vi "EstimateAbsoluteOrientation2D.vi"(5 "Point Set Weights (Default: Empty - Equal Weights)":dbl[](array[numeric]), 7 "Termination Criterion in":refnum<class "Termination Criteria.lvclass">, 8 "error in":errorcluster, 10 "Reference Point Set (Default - Use First  Set of Corresponding Points Array)":map{i32, T1}(c390), 11 "Image Point Sets":map{i32, T1}[](array[numeric])) -> (0 "error out":errorcluster, 1 "T Vectors":T1[](array[typedef]), 2 "R Matricies":dbl[][][](array[numeric]), 3 "Optimized Points":map{i32, T1}(c390), 4 "Scale Values":dbl[](array[numeric]))   [LabVIEW 2020, in "ar.lvlib"]
doc: "Estimate the Absolute Orientation of multiple views of the same 2D Point Set. \n\nThis can be used to combine multiple samples of the same object point sets to reduce mean square errors in an absolute set of positions."
uses:
  ar.lvlib
  common/Termination Criteria/Termination Criteria.lvclass
  common/Image Point (Float).ctl
  common/Termination Criteria/Termination Criteria.lvclass/Termination Criteria.ctl
  808428ba-76ae-4f0f-a703-b2147cff2032.vi
  EstimateTransformParametersBetweenPointSets.vi
  OptimizePointSetFromPointSetCorrespondenceTransforms.vi
  Dimensions.vi
  common/Termination Criteria/Get Values.vi
  808428ba-76ae-4f0f-a703-b2147cff2032.vi/b761b6b4-53cc-4592-85b1-23315e9e6a73.vi
  SubtractMeanFromPoints.vi
  CovarianceofPointSetsA&B.vi
  DecomposeCovarianceOfPointSetsA&B.vi
  <vilib>/Analysis/baseanly.llb/A x Vector.vi
  <vilib>/Analysis/baseanly.llb/A x B.vi
  <vilib>/Analysis/baseanly.llb/Mean.vi
  <vilib>/Analysis/baseanly.llb/Mean (DBL).vi
  <vilib>/Analysis/baseanly.llb/Real A x B.vi
  <vilib>/Analysis/baseanly.llb/Determinant.vi
  <vilib>/Analysis/baseanly.llb/Real Determinant.vi
  SVDForPointSetCovarainces.vi
  <vilib>/Analysis/_algsub.llb/Matrix Rank.vi
  <vilib>/Analysis/_algsub.llb/Real Matrix Rank.vi
  <vilib>/Analysis/_algsub.llb/Trace.vi
  <vilib>/Analysis/_algsub.llb/Real Matrix Trace.vi
  <vilib>/Utility/error.llb/Error Cluster From Error Code.vi
  <vilib>/Analysis/7linalg.llb/Create Special Real Matrix.vi
  <vilib>/Analysis/Matrix/Numeric/Conversions/Array To Matrix - RA2.vi
  <vilib>/Analysis/7linalg.llb/SVD Decomposition.vi
  <vilib>/Analysis/7linalg.llb/Real SVD Decomposition.vi
  <vilib>/Analysis/7linalg.llb/Create Special Matrix.vi
  <vilib>/Analysis/Matrix/Numeric/Multiply/Multiply - RM,R.vi
  common/common.lvlib
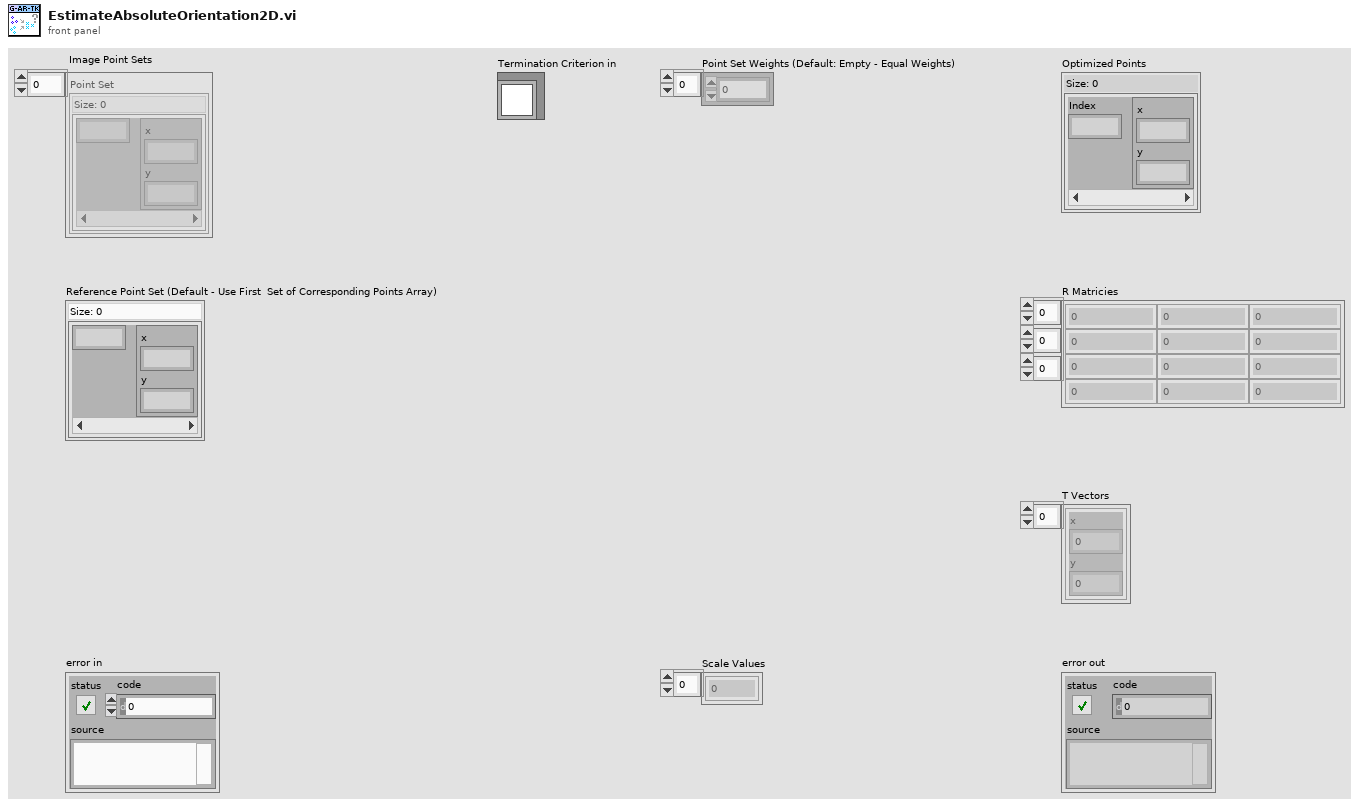
[diagram p1: front panel]
types:
  T1 = typedef "common.lvlib/Image Point (Float).ctl" = cluster{"x":dbl, "y":dbl}
  T2 = typedef "ar.lvlib/PointSet.ctl" = dbl[][]
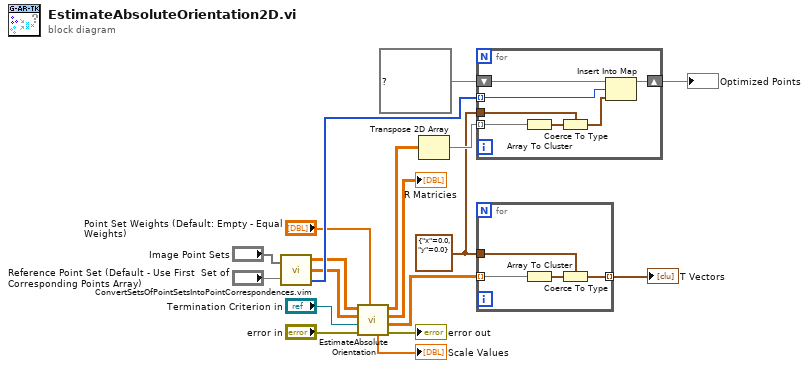
[diagram p0: block diagram]
diagram:
  w4 = T1 {"x"=0.0, "y"=0.0} ("Point")
  n1 = call "ConvertSetsOfPointSetsIntoPointCorrespondences.vim"("Image Point Sets"="Image Point Sets", "Reference Point Set"="Reference Point Set (Default - Use First  Set of Corresponding Points Array)") -> ("Coresponding Point Sets"=w6:dbl[][][], "Reference Points"=w7:dbl[][], "Indicies"=w8:i32[])  [unwired: 1 in]
  n2 = call "EstimateAbsoluteOrientation.vi"("Point Set Weights"="Point Set Weights (Default: Empty - Equal Weights)", "error in"="error in", "Termination Criterion in"="Termination Criterion in", "Reference Object Point"=w7, "Corresponding Object Points Array"=w6) -> ("error out"=→"error out":errorcluster, "T Vectors"=w3:dbl[][], "R Matricies"=→"R Matricies":dbl[][][], "Optimized Point Set"=w2:T2, "Scale Values"=→"Scale Values":dbl[])  [unwired: 2 in]
  n3 = Transpose 2D Array(2D array=w2) -> (transposed array=w5:T2)
  n4 = for {
    tunnel: w5 -> [w25] mode=indexing
    tunnel: w4 -> [w23]
    tunnel: w8 -> [w22] mode=indexing
    shift-right: [w20] -> w10
    shift-left: map{i32, T1} {} ("Size: 0") -> [w19]
    n5 = Array To Cluster(array=w25) -> (cluster=w24:cluster{"[0]":dbl, "[1]":dbl})
    n6 = Coerce To Type(0:w24, 1:w23) -> (2:w21:T1)
    n7 = Insert Into Map(map in=w19, key=w22, value=w21) -> (map out=w20:map{i32, T1})  [unwired: 2 out]
  }
  "Optimized Points" <- w10
  n8 = for {
    tunnel: w3 -> [w29] mode=indexing
    tunnel: w4 -> [w27]
    tunnel: [w26] -> w15 mode=indexing
    n9 = Array To Cluster(array=w29) -> (cluster=w28:cluster{"T Vectors[0]":dbl, "T Vectors[1]":dbl})
    n10 = Coerce To Type(0:w28, 1:w27) -> (2:w26:T1)
  }
  "T Vectors" <- w15
